vi "niFPGA Threshold Crossing.vi"   [LabVIEW 2017]
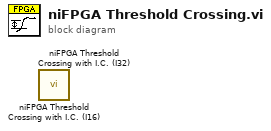
[diagram p0: block diagram]
diagram:
  n1 = call <vilib>:"niFPGA Threshold Crossing with I.C. (I16).vi"() -> ()  [unwired: 10 in, 2 out]
  n2 = call <vilib>:"niFPGA Threshold Crossing with I.C. (I32).vi"() -> ()  [unwired: 10 in, 2 out]
